vi "array.vi"() -> ()   [LabVIEW 2019]
uses:
  <vilib>/Analysis/Matrix/Datatypes/RealMatrix.ctl
  <vilib>/Analysis/Matrix/Numeric/Conversions/Array To Matrix - RA.vi
  <vilib>/Analysis/Matrix/Numeric/Add/Add (Elementwise) - RM,R.vi
  <vilib>/Analysis/Matrix/NI_Matrix.lvlib
panel:
  out "A + c":T1
  out "appended array":i32[](array[numeric])
  out "initialized array 2":bool[](array[boolean])
  out "initialized array":dbl[](array[numeric])
  out "output array 2":i32[](array[numeric])
  out "output array":i32[](array[numeric])
  out "element":i32
  out "size(s)":i32
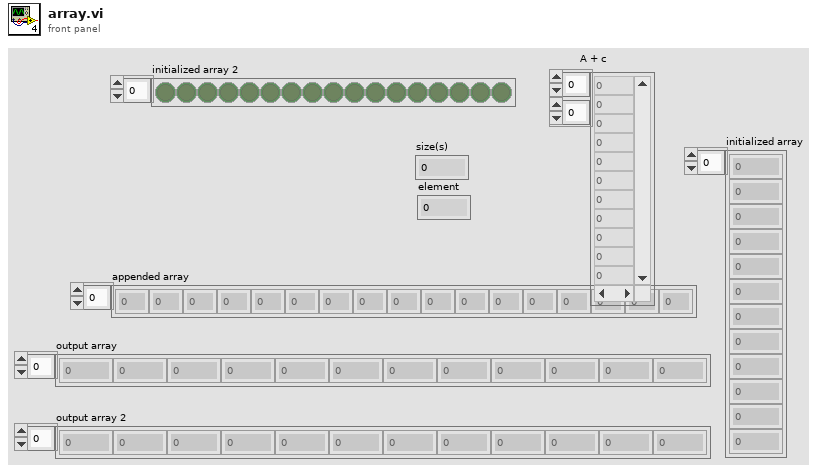
[diagram p1: front panel]
types:
  T1 = typedef "NI_Matrix.lvlib/RealMatrix.ctl" = dbl[][]
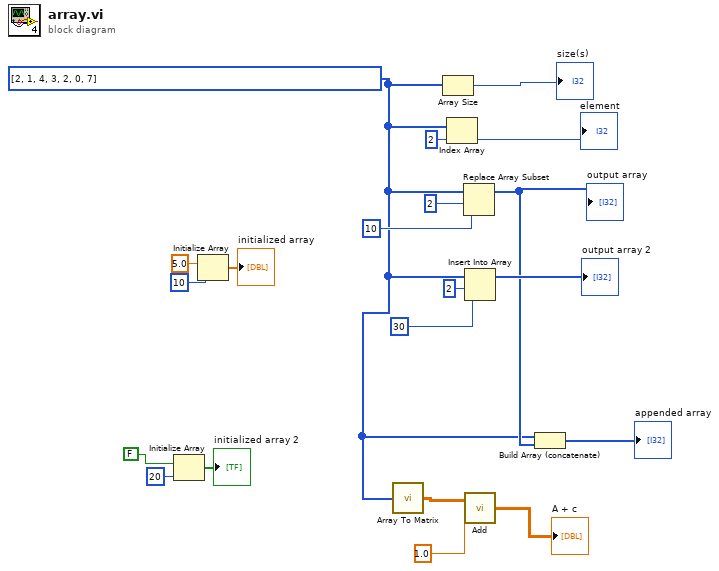
[diagram p0: block diagram]
diagram:
  w4 = i32[] [2, 1, 4, 3, 2, 0, 7]
  n1 = Initialize Array(FALSE, 20 ("dimension size")) -> (→"initialized array 2":bool[])
  n2 = Initialize Array(5.0 ("element"), 10 ("dimension size")) -> (→"initialized array":dbl[])
  n3 = call-poly <vilib>:"Array To Matrix.vi"("Real 1D Array"=w4) -> ("Real Matrix (Column Vector)"=w3:T1)
  n4 = Array Size(array=w4) -> (size(s)=→"size(s)":i32)
  n5 = Index Array(array=w4, index=2) -> (element=→"element":i32)
  n6 = Replace Array Subset(array=w4, new element=10 ("new element/subarray"), index=2) -> (w6:i32[])
  "output array" <- w6
  n7 = Insert Into Array(array=w4, index=2, new element=30 ("new element/subarray")) -> (→"output array 2":i32[])
  n8 = call-poly <vilib>:"Add.vi"("Real Scalar c"=1.0, "Real Matrix A"=w3) -> ("A + c"=→"A + c":T1)
  n9 = Build Array (concatenate)(w4, w6) -> (→"appended array":i32[])
